vi "Pop Standard Header.vi"(8 "error in (no error)":errorcluster, 11 "Header in":refnum<class "Header.lvclass">) -> (0 "error out":errorcluster, 2 "Std Header":string, 3 "Header out":refnum<class "Header.lvclass">)   [LabVIEW 2018, in "Header.lvclass"]
uses:
  Header.lvclass
  Header.lvclass/Header.ctl
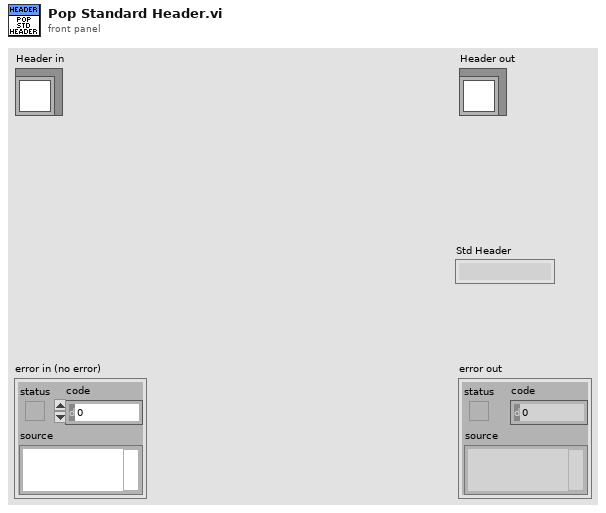
[diagram p1: front panel]
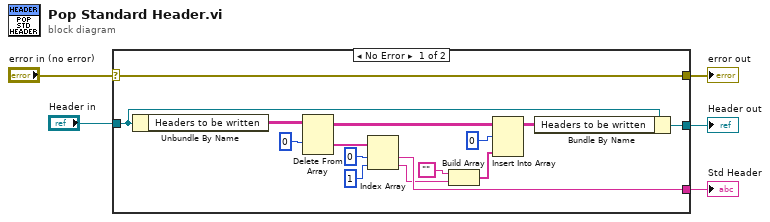
[diagram p0: block diagram]
diagram:
  n1 = case shown="No Error" "error in (no error)" {
    selector: "error in (no error)" -> [w20 w22]
    tunnel: [w20 w22] -> w4
    tunnel: [w16 w21] -> w2
    tunnel: "Header in" -> [w17 w21]
    tunnel: [w11 _] -> w1
    frame No Error {
      n2 = Unbundle By Name(w17) -> ("Headers to be written"=w19:string[][])
      n3 = Delete From Array(array=w19, index (row)=0) -> (deleted portion=w12:string[], array with subset deleted=w15:string[][])  [unwired: 2 in]
      n4 = Index Array(array=w12, index #1=0 ("index (row)"), index #2=1 ("index (row)")) -> (element #1=w11:string, element #2=w8:string)
      n5 = Build Array("", w8) -> (w6:string[])
      n6 = Insert Into Array(array=w15, index (row)=0, new element=w6) -> (w14:string[][])  [unwired: 1 in]
      n7 = Bundle By Name(cluster=w17, "Headers to be written"=w14) -> (w16:refnum<class "Header.lvclass">)
    }
    frame Error {
    }
  }
  "error out" <- w4
  "Header out" <- w2
  "Std Header" <- w1
